vi "Read_file_to_2_1D_arrays.vi"(7 "delimiter (space)":string=" ", 8 "error in (no error)":errorcluster, 11 "Path":path) -> (0 "error out":errorcluster, 3 "ProgramData":T1)   [LabVIEW 2020]
doc: "This VI read dictionary data from file located in <b>Path</b>. Words from dictionary are seperated by specified <b>delimeter(space)</b>. VI returns English Words, Polish Words and Numbers of Pairs from dictionary, all this output data is stored in cluster <b>#typedef_ProgramData</b>."
uses:
  #typedef_Program_Data.ctl
  #typedef_English_Teacher_States.ctl
  #typedef_WordsActions.ctl
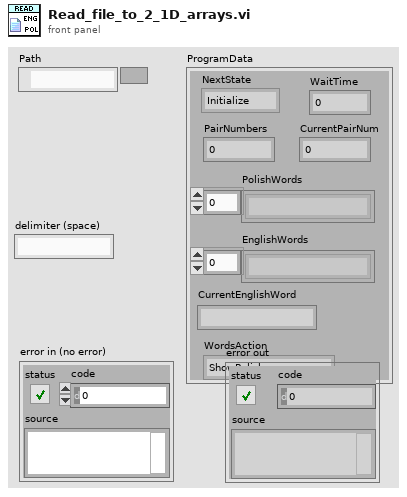
[diagram p1: front panel]
types:
  T1 = typedef "#typedef_Program_Data.ctl" = cluster{"WaitTime":dbl, "PolishWords":string[], "EnglishWords":string[], "PairNumbers":i32, "NextState":T2, "WordsAction":T3, "CurrentPairNum":i32, "CurrentEnglishWord":string}
  T2 = typedef "#typedef_English_Teacher_States.ctl" = enum16{"Initialize", "Idle", "Learning_1", "Learning_2", "Learning_3", "Test_1", "Test_2", "Test_3", "Test_4", "Stop", "Exit"}
  T3 = typedef "#typedef_WordsActions.ctl" = enum16{"ShowPolish", "ShowEnglish", "ShowBoth", "ShowNone"}
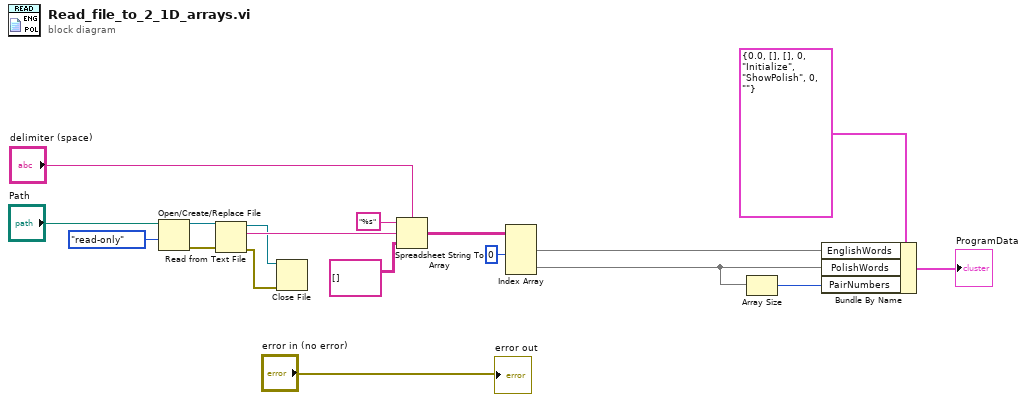
[diagram p0: block diagram]
diagram:
  n1 = Open/Create/Replace File(file path (use dialog)="Path", access (0:read/write)=enum16{"read/write", "read-only", "write-only"}."read-only") -> (refnum out=w4:refnum<file>, error out=w5:errorcluster)  [unwired: 4 in, 1 out]
  n2 = Read from Text File(file (use dialog)=w4, error in=w5) -> (refnum out=w7:refnum<file>, text=w10:string, error out=w8:errorcluster)  [unwired: 2 in, 1 out]
  n3 = Close File(refnum=w7, error in=w8) -> ()  [unwired: 2 out]
  n4 = Spreadsheet String To Array(delimiter (Tab)="delimiter (space)", format string="%s", spreadsheet string=w10, array type (2D Dbl)=string[][] []) -> (array=w14:string[][])
  n5 = Index Array(array=w14, index (col) #1=0 ("disabled index (col)")) -> (element #1=w17:string[], element #2=w18:string[])  [unwired: 3 in]
  n6 = Array Size(array=w18) -> (size(s)=w1:i32)
  n7 = Bundle By Name(cluster=T1 {"WaitTime"=0.0, "PolishWords"=[], "EnglishWords"=[], "PairNumbers"=0, "NextState"=enum."Initialize", "WordsAction"=enum."ShowPolish", "CurrentPairNum"=0, "CurrentEnglishWord"=""} ("ProgramData"), "EnglishWords"=w17, "PolishWords"=w18, "PairNumbers"=w1) -> (→"ProgramData":T1)
  "error out" <- "error in (no error)"
